vi "ellipse model.vi"(3 "output control":T1, 4 "data":variant, 5 "X":dbl[](array[numeric]), 6 "a":dbl[](array[numeric])) -> (0 "error out":errorcluster, 1 "f'(X,a)":dbl[][](array[numeric]), 2 "f(X,a)":dbl[](array[numeric]))   [LabVIEW 2023]
doc: "Implements an ellipse model function to be passed to the Nonlinear Curve Fit.vi."
uses:
  <vilib>/gmath/NumericalOptimization/LM_output select.ctl
  <vilib>/gmath/NI_Gmath.lvlib
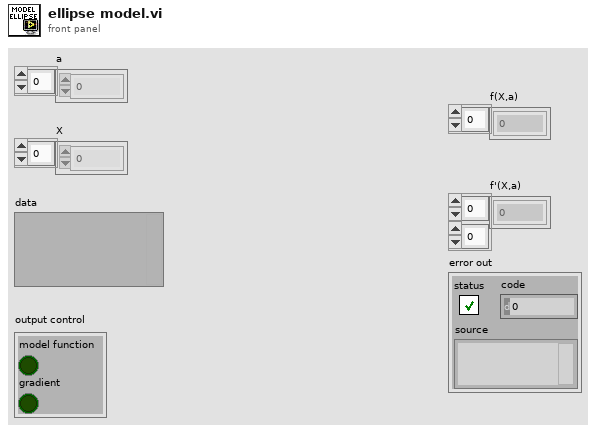
[diagram p1: front panel]
types:
  T1 = typedef "NI_Gmath.lvlib/LM_output select.ctl" = cluster{"model function":bool, "gradient":bool}
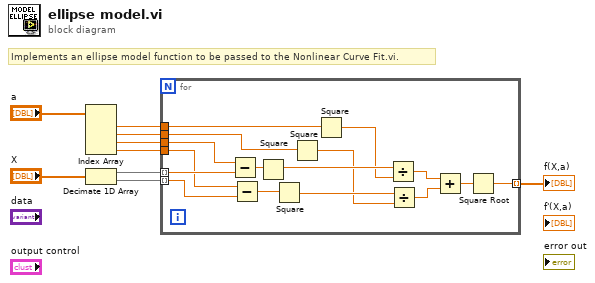
[diagram p0: block diagram]
diagram:
  # "Implements an ellipse model function to be passed to the Nonlinear Curve Fit.vi."
  n1 = Index Array(array="a") -> (element #1=w7:dbl, element #2=w6:dbl, element #3=w5:dbl, element #4=w1:dbl)  [unwired: 4 in]
  n2 = Decimate 1D Array("X") -> (w3:dbl[], w2:dbl[])
  n3 = for {
    tunnel: w3 -> [w25] mode=indexing
    tunnel: w7 -> [w22]
    tunnel: w6 -> [w16]
    tunnel: w5 -> [w18]
    tunnel: [w19] -> w4 mode=indexing
    tunnel: w2 -> [w20] mode=indexing
    tunnel: w1 -> [w17]
    n4 = Subtract(x=w18, y=w25) -> (x-y=w23:dbl)
    n5 = Subtract(x=w17, y=w20) -> (x-y=w24:dbl)
    n6 = Square(x=w23) -> (x^2=w15:dbl)
    n7 = Square(x=w24) -> (x^2=w14:dbl)
    n8 = Square(x=w16) -> (x^2=w12:dbl)
    n9 = Square(x=w22) -> (x^2=w13:dbl)
    n10 = Divide(x=w15, y=w13) -> (x/y=w11:dbl)
    n11 = Divide(x=w14, y=w12) -> (x/y=w10:dbl)
    n12 = Add(x=w11, y=w10) -> (x+y=w21:dbl)
    n13 = Square Root(x=w21) -> (sqrt(x)=w19:dbl)
  }
  "f(X,a)" <- w4
